vi "Min Read Array.vi"(8 "error in":errorcluster, 11 "Min Limit in":refnum<class "Limit.lvclass">) -> (0 "error out":errorcluster, 1 "Changed or First Call?":bool, 2 "Current Min SP":dbl[](array[numeric]), 3 "Min Limit out":refnum<class "Limit.lvclass">)   [LabVIEW 2023, in "Limit.lvclass"]
uses:
  Limit.lvclass
  266b4bec-33ea-4549-af17-4c009f6fd026.vi
  <vilib>/ADAS Replay HIL/Channels/Tag Wrapper/Tag Wrapper.lvlib
  <vilib>/ADAS Replay HIL/Channels/Tag Wrapper/Polymorphic/Read Channel (Double).vi
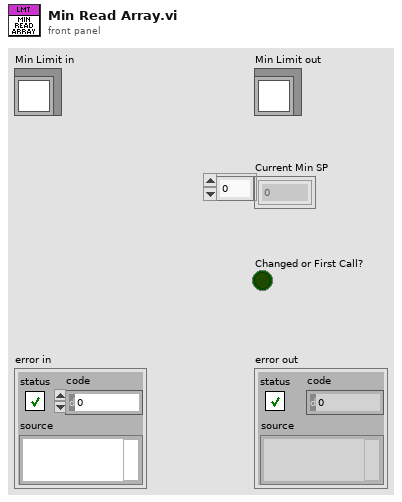
[diagram p1: front panel]
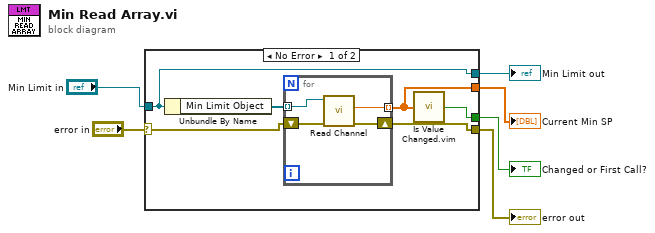
[diagram p0: block diagram]
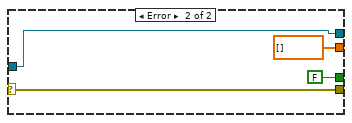
[diagram p2: hidden frame]
diagram:
  n1 = case shown="No Error" "error in" {
    selector: "error in" -> [w10 w20]
    tunnel: [w9 w20] -> w1
    tunnel: [w12 w19] -> w4
    tunnel: "Min Limit in" -> [w12 w19]
    tunnel: [w8 dbl[] []] -> w3
    tunnel: [w7 FALSE ("changed or first call?")] -> w2
    frame No Error {
      n2 = Unbundle By Name(w12) -> ("Min Limit Object"=w11:refnum<k21>[])
      n3 = for {
        tunnel: w11 -> [w16] mode=indexing
        tunnel: [w13] -> w8 mode=indexing
        shift-right: [w14] -> w9
        shift-left: w10 -> [w15]
        n4 = call-poly <vilib>:"Read Channel.vi"("error in"=w15, "ADAS HIL Channel in"=w16) -> ("error out"=w14:errorcluster, "Value out"=w13:dbl)  [unwired: 6 in, 2 out]
      }
      n5 = call "Is Value Changed.vim"("value"=w8) -> ("changed or first call?"=w7:bool)
    }
    frame Error {
    }
  }
  "error out" <- w1
  "Changed or First Call?" <- w2
  "Current Min SP" <- w3
  "Min Limit out" <- w4
